vi "AES Generate Key.vi"(8 "error in (no error)":errorcluster, 11 "AES in":refnum<class "AES.lvclass">) -> (0 "error out":errorcluster, 1 "IV":u8[](array[numeric]), 2 "Key":u8[](array[numeric]), 3 "AES out":refnum<class "AES.lvclass">)   [LabVIEW 2021, in "AES.lvclass"]
uses:
  AES.lvclass
  AES.lvclass/AES.ctl
  System.Core
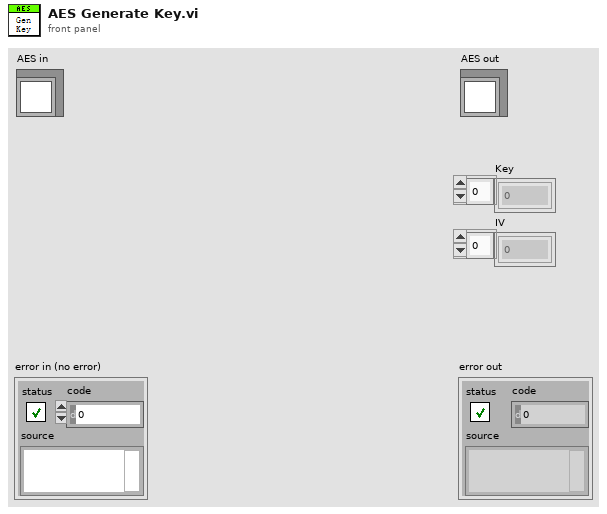
[diagram p1: front panel]
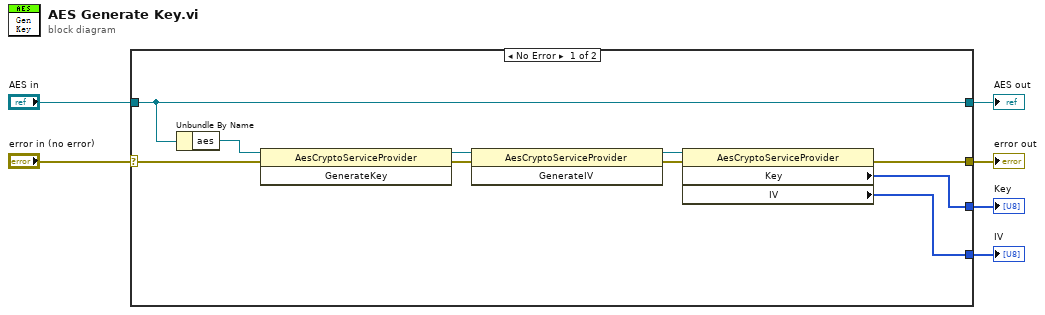
[diagram p0: block diagram]
diagram:
  n1 = case shown="No Error" "error in (no error)" {
    selector: "error in (no error)" -> [w13 w18]
    tunnel: [w9 w18] -> w5
    tunnel: [w16 w17] -> w3
    tunnel: "AES in" -> [w16 w17]
    tunnel: [w8 _] -> w2
    tunnel: [w7 _] -> w1
    frame No Error {
      n2 = Unbundle By Name(w16) -> ("aes"=w12:refnum<k24>)
      n3 = invoke class="AesCryptoServiceProvider" method="GenerateKey"(reference=w12, error in=w13) -> (reference out=w15:refnum<k24>, error out=w14:errorcluster)  [unwired: 1 in, 1 out]
      n4 = invoke class="AesCryptoServiceProvider" method="GenerateIV"(reference=w15, error in=w14) -> (reference out=w10:refnum<k24>, error out=w11:errorcluster)  [unwired: 1 in, 1 out]
      n5 = property class="AesCryptoServiceProvider"(reference=w10, error in=w11) -> (error out=w9:errorcluster, "Key"=w8:u8[], "IV"=w7:u8[])  [unwired: 1 out]
    }
    frame Error {
    }
  }
  "error out" <- w5
  "AES out" <- w3
  "Key" <- w2
  "IV" <- w1
